vi "test_MonoOpenAndClose.vi"(7 "Test should pass":bool=TRUE, 8 "error in":errorcluster, 9 "tear down connection":bool=TRUE, 10 "set-up a connection":bool=TRUE, 11 "device selection":enum16{"monochromator", "CCD", "SCD"}(ring)) -> (0 "error out":errorcluster, 2 "log-file path":path)   [LabVIEW 2023]
uses:
  <vilib>/addons/_JKI Toolkits/Caraya/classes/Assert/Assert Equal Value and Type_Variant.vi
  <vilib>/addons/_JKI Toolkits/Caraya/classes/Assert/Assert Not Error.vi
  Classes/GenericDevice/GenericDevice.lvclass
  <vilib>/addons/_JKI Toolkits/Caraya/classes/Test/Test.lvclass
  <vilib>/addons/_JKI Toolkits/Caraya/classes/Assert/Assert.lvclass
  <vilib>/Hampel Software Engineering/HSE Logger/hse-logger.lvlib
panel:
  # "Connector Pane"
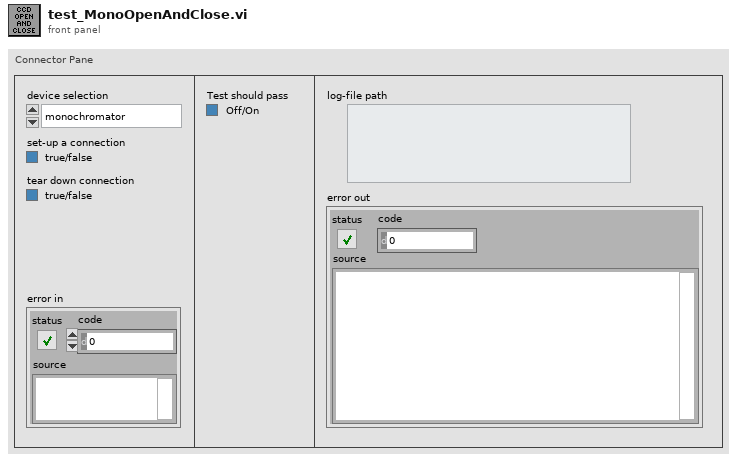
[diagram p1: front panel]
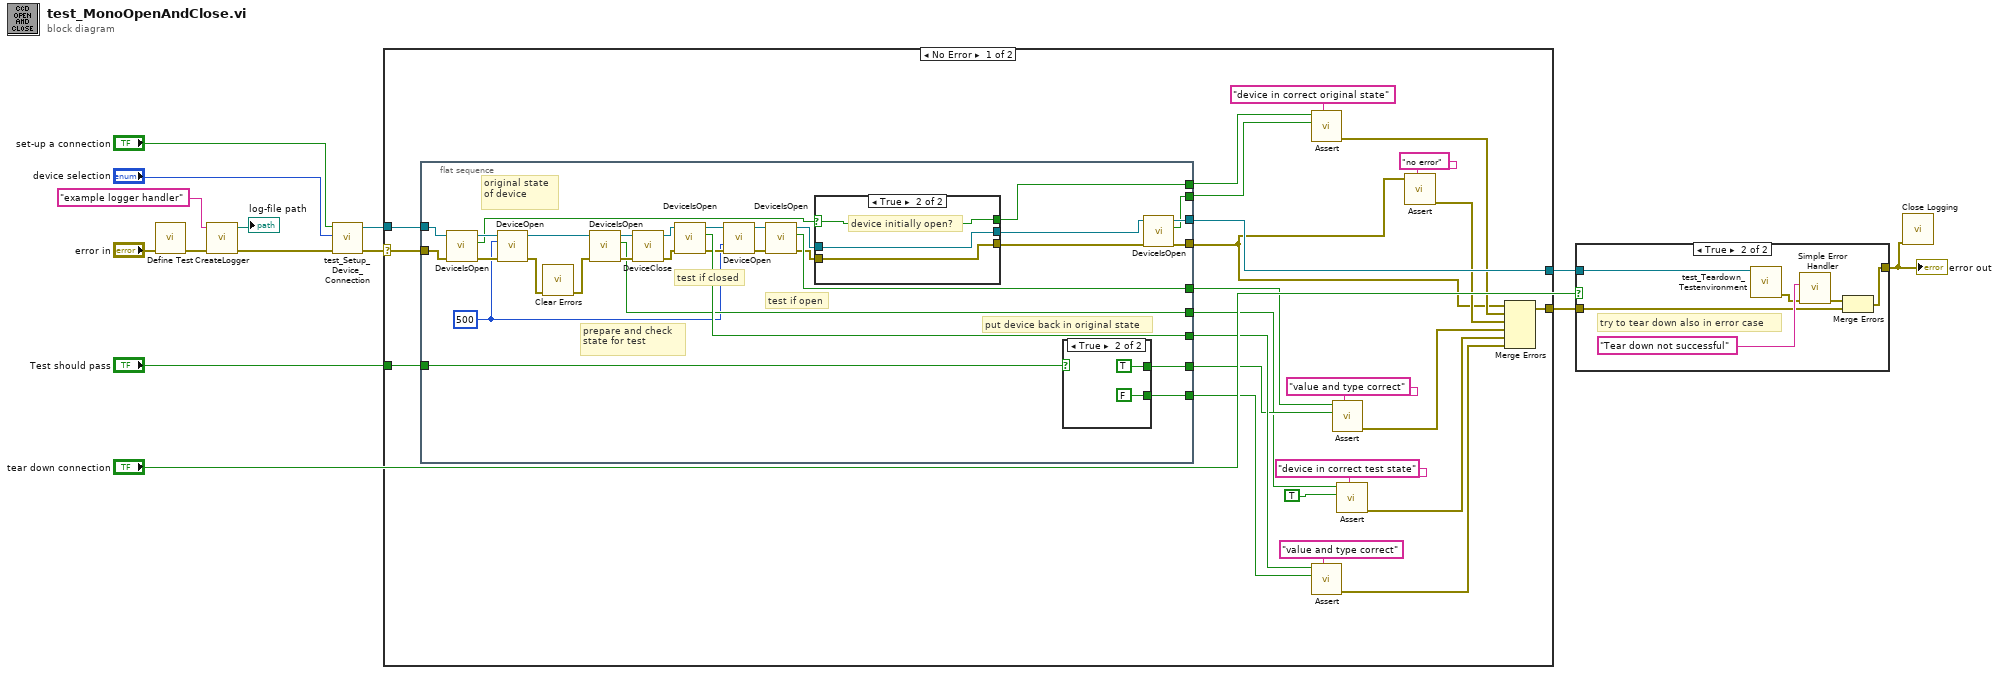
[diagram p0: block diagram]
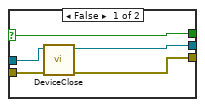
[diagram p2: hidden frame]
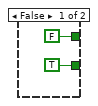
[diagram p3: hidden frame]
diagram:
  n1 = call <vilib>:"Define Test.vi"("error in (no error)"="error in") -> ("error out"=w5:errorcluster)  [unwired: 9 in, 1 out]
  n2 = call "CreateLogger.vi"("error in (no error)"=w5, "Handler Name"="example logger handler") -> ("error out"=w3:errorcluster, "log-file path"=→"log-file path":path)  [unwired: 8 in]
  n3 = call "test_Setup_Device_Connection.vi"("error in (no error)"=w3, "device selection"="device selection", "set-up a connection"="set-up a connection") -> ("error out"=w6:errorcluster, "GenericDevice.lvclass"=w9:refnum<class "GenericDevice.lvclass">)  [unwired: 7 in]
  n4 = case shown="No Error" w6 {
    selector: w6 -> [w15 w83]
    tunnel: "Test should pass" -> [w34 _]
    tunnel: [w33 w82] -> w10
    tunnel: w9 -> [w22 w82]
    tunnel: [w16 w83] -> w7
    frame No Error {
      n5 = flat-sequence {
        tunnel: w15 -> [w68]
        tunnel: [w44] -> w17
        tunnel: w34 -> [w69]
        tunnel: [w48] -> w33
        tunnel: [w61] -> w32
        tunnel: [w60] -> w31
        tunnel: [w59] -> w30
        tunnel: [w58] -> w29
        tunnel: [w57] -> w27
        tunnel: [w50] -> w24
        tunnel: [w47] -> w23
        tunnel: w22 -> [w40]
        frame #0 {
          w39 = 500 ("Delay between send and receive [ms]")
          # "put device back in original state"
          # "test if open"
          # "test if closed"
          # "original state of device"
          # "prepare and check state for test"
          n6 = call-dynamic "DeviceIsOpen.vi"("error in (no error)"=w68, "GenericDevice in"=w40) -> ("error out"=w43:errorcluster, "device is open?"=w56:bool, "GenericDevice out"=w67:refnum<class "GenericDevice.lvclass">)  [unwired: 6 in, 1 out]
          n7 = call-dynamic "DeviceOpen.vi"("error in (no error)"=w43, "Delay between send and receive [ms]"=w39, "GenericDevice in"=w67) -> ("error out"=w42:errorcluster, "GenericDevice out"=w66:refnum<class "GenericDevice.lvclass">)  [unwired: 5 in, 2 out]
          n8 = call <vilib>:"Clear Errors.vi"("error in (no error)"=w42) -> ("error out"=w41:errorcluster)  [unwired: 5 in, 1 out]
          n9 = call-dynamic "DeviceIsOpen.vi"("error in (no error)"=w41, "GenericDevice in"=w66) -> ("error out"=w62:errorcluster, "device is open?"=w57:bool, "GenericDevice out"=w65:refnum<class "GenericDevice.lvclass">)  [unwired: 6 in, 1 out]
          n10 = call-dynamic "DeviceClose.vi"("error in (no error)"=w62, "GenericDevice in"=w65) -> ("error out"=w63:errorcluster, "GenericDevice out"=w64:refnum<class "GenericDevice.lvclass">)  [unwired: 5 in, 3 out]
          n11 = call-dynamic "DeviceIsOpen.vi"("error in (no error)"=w63, "GenericDevice in"=w64) -> ("error out"=w52:errorcluster, "device is open?"=w61:bool, "GenericDevice out"=w54:refnum<class "GenericDevice.lvclass">)  [unwired: 6 in, 1 out]
          n12 = call-dynamic "DeviceOpen.vi"("error in (no error)"=w52, "Delay between send and receive [ms]"=w39, "GenericDevice in"=w54) -> ("error out"=w51:errorcluster, "GenericDevice out"=w53:refnum<class "GenericDevice.lvclass">)  [unwired: 5 in, 2 out]
          n13 = call-dynamic "DeviceIsOpen.vi"("error in (no error)"=w51, "GenericDevice in"=w53) -> ("error out"=w46:errorcluster, "device is open?"=w59:bool, "GenericDevice out"=w55:refnum<class "GenericDevice.lvclass">)  [unwired: 6 in, 1 out]
          n14 = case shown="True" w56 {
            selector: w56 -> [w72 w75]
            tunnel: w55 -> [w74 w77]
            tunnel: [w73 w77] -> w49
            tunnel: [w72 w75] -> w50
            tunnel: w46 -> [w71 w76]
            tunnel: [w70 w76] -> w45
            frame False {
              n15 = call-dynamic "DeviceClose.vi"("error in (no error)"=w71, "GenericDevice in"=w74) -> ("error out"=w70:errorcluster, "GenericDevice out"=w73:refnum<class "GenericDevice.lvclass">)  [unwired: 5 in, 3 out]
            }
            frame True {
              # "device initially open?"
            }
          }
          n16 = case shown="True" w69 {
            tunnel: [TRUE ("device is open?") FALSE ("device is open?")] -> w60
            tunnel: [FALSE ("device is open?") TRUE ("device is open?")] -> w58
            frame False {
            }
            frame True {
            }
          }
          n17 = call-dynamic "DeviceIsOpen.vi"("error in (no error)"=w45, "GenericDevice in"=w49) -> ("error out"=w44:errorcluster, "device is open?"=w47:bool, "GenericDevice out"=w48:refnum<class "GenericDevice.lvclass">)  [unwired: 6 in, 1 out]
        }
      }
      n18 = call-poly <vilib>:"Assert.vi"("Label"="device in correct original state" ("Label (VI Title)"), "Y"=w23, "X"=w24) -> ("error out"=w18:errorcluster)  [unwired: 7 in, 1 out]
      n19 = call-poly <vilib>:"Assert.vi"("Label"="value and type correct" ("Label (VI Title)"), "Y"=w31, "X"=w32) -> ("error out"=w20:errorcluster)  [unwired: 7 in, 1 out]
      n20 = call-poly <vilib>:"Assert.vi"("Label"="value and type correct" ("Label (VI Title)"), "Y"=w29, "X"=w30) -> ("error out"=w37:errorcluster)  [unwired: 7 in, 1 out]
      n21 = call-poly <vilib>:"Assert.vi"("Label"="device in correct test state" ("Label (VI Title)"), "Y"=TRUE ("device is open?"), "X"=w27) -> ("error out"=w21:errorcluster)  [unwired: 7 in, 1 out]
      n22 = call-poly <vilib>:"Assert.vi"("Label"="no error" ("Label (VI Title)"), "Not Error?"=w17) -> ("error out"=w19:errorcluster)  [unwired: 8 in, 1 out]
      n23 = Merge Errors(w17, w18, w19, w37, w21, w20) -> (w16:errorcluster)
    }
    frame Error {
    }
  }
  n24 = case shown="True" "tear down connection" {
    tunnel: w10 -> [_ w89]
    tunnel: [w84 w85] -> w1
    tunnel: w7 -> [w84 w86]
    frame False {
    }
    frame True {
      # "try to tear down also in error case"
      n25 = call "test_Teardown_Testenvironment.vi"("GenericDevice.lvclass"=w89) -> ("error out"=w88:errorcluster)  [unwired: 9 in, 1 out]
      n26 = call <vilib>:"Simple Error Handler.vi"("error source (\" \")"="Tear down not successful" ("error source (\" \")"), "error in (no error)"=w88) -> ("error out"=w87:errorcluster)  [unwired: 3 in, 4 out]
      n27 = Merge Errors(w87, w86) -> (w85:errorcluster)
    }
  }
  "error out" <- w1
  n28 = call <vilib>:"Close Logging.vi"("error in"=w1) -> ()  [unwired: 10 in, 1 out]
